vi "Add Elements to MeasLink UI.vi"(11 "error in (no error)":errorcluster) -> (15 "error out":errorcluster)   [LabVIEW 2021, in "Migrator.lvlib"]
uses:
  Migrator.lvlib
  Path Functions/Path Functions.lvlib
  Migrator Reusables/Migrator Reusables.lvlib
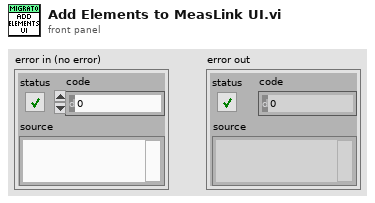
[diagram p1: front panel]
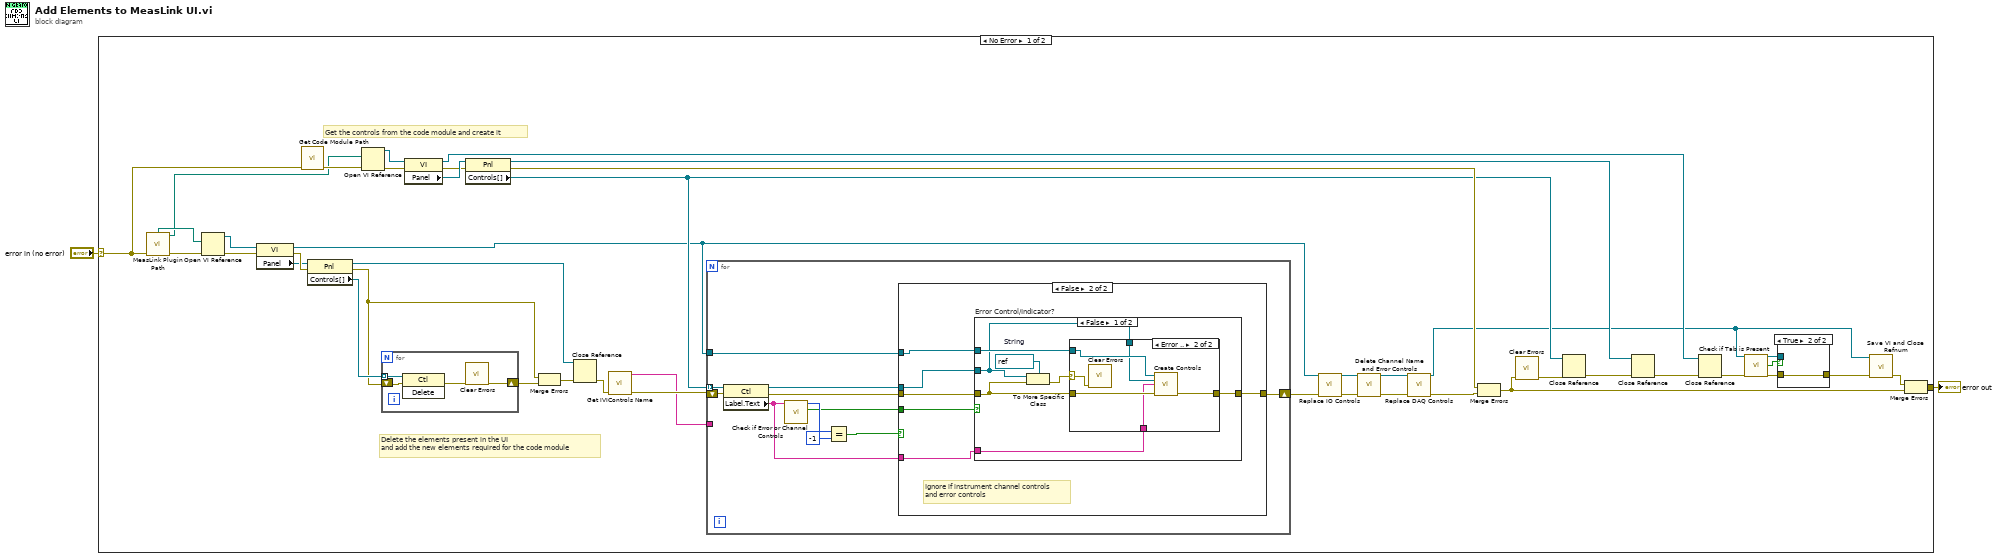
[diagram p0: block diagram]
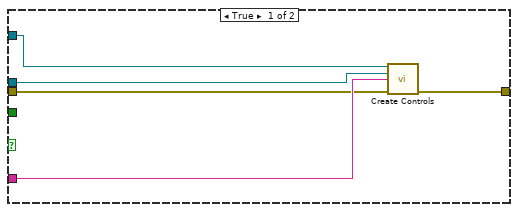
[diagram p2: hidden frame]
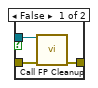
[diagram p5: hidden frame]
diagram:
  n1 = case shown="No Error" "error in (no error)" {
    selector: "error in (no error)" -> [w31 w92]
    tunnel: [w36 w92] -> w2
    frame No Error {
      # "Get the controls from the code module and create it"
      # "Delete the elements present in the UI\nand add the new elements required for the code module"
      n2 = call "MeasLink Plugin Path.vi"("error in (no error)"=w31) -> ("Measurement UI"=w33:path, "New Code Module"=w11:path, "error out"=w46:errorcluster)  [unwired: 2 in, 10 out]
      n3 = Open VI Reference(vi path=w33, error in (no error)=w46) -> (vi reference=w21:refnum<vi>, error out=w45:errorcluster)  [unwired: 4 in]
      n4 = property class="VI"(reference=w21, error in=w45) -> (reference out=w25:refnum<vi>, error out=w44:errorcluster, "Panel"=w27:refnum<vi>)
      n5 = call "Get Code Module Path.vi"("error in (no error)"=w31) -> ("error out"=w30:errorcluster)  [unwired: 13 in, 1 out]
      n6 = property class="Pnl"(reference=w27, error in=w44) -> (reference out=w26:refnum<vi>, error out=w12:errorcluster, "Controls[]"=w43:refnum<vi>[])
      n7 = Open VI Reference(vi path=w11, error in (no error)=w30) -> (vi reference=w18:refnum<vi>, error out=w38:errorcluster)  [unwired: 4 in]
      n8 = for {
        tunnel: w43 -> [w50] mode=indexing
        shift-right: [w47] -> w42
        shift-left: w12 -> [w49]
        n9 = invoke class="Ctl" method="Delete"(reference=w50, error in=w49) -> (error out=w48:errorcluster)  [unwired: 1 in, 2 out]
        n10 = call <vilib>:"Clear Errors.vi"("error in (no error)"=w48) -> ("error out"=w47:errorcluster)  [unwired: 5 in, 1 out]
      }
      n11 = property class="VI"(reference=w18, error in=w38) -> (reference out=w17:refnum<vi>, error out=w37:errorcluster, "Panel"=w39:refnum<vi>)
      n12 = property class="Pnl"(reference=w39, error in=w37) -> (reference out=w16:refnum<vi>, error out=w41:errorcluster, "Controls[]"=w40:refnum<vi>[])
      n13 = Merge Errors(w12, w42) -> (w13:errorcluster)
      n14 = Close Reference(reference=w26, error in (no error)=w13) -> (error out=w20:errorcluster)
      n15 = call "Get IVIControls Name.vi"("error in (no error)"=w20) -> ("Control Names Out"=w28:string[], "error out"=w29:errorcluster)  [unwired: 12 in, 1 out]
      n16 = for {
        tunnel: w25 -> [w61]
        tunnel: w40 -> [w59] mode=indexing
        shift-right: [w60] -> w24
        shift-left: w29 -> [w58]
        tunnel: w28 -> [_]
        n17 = property class="Ctl"(reference=w59, error in=w58) -> (reference out=w56:refnum<vi>, error out=w55:errorcluster, "Label.Text"=w57:string)
        n18 = call "Check if Error or Channel Controls.vi"("Label.Text"=w57) -> ("Error?"=w51:bool, "offset past match"=w54:i32)  [unwired: 9 in]
        n19 = Equal?(x=w54, y=-1) -> (x = y?=w52:bool)
        n20 = case shown="False" w52 {
          tunnel: w61 -> [w66 w69]
          tunnel: [w65 w67] -> w60
          tunnel: w56 -> [w63 w72]
          tunnel: w55 -> [w62 w71]
          tunnel: w57 -> [w64 w68]
          tunnel: w51 -> [_ w70]
          frame True {
            n21 = call "Create Controls.vi"("VI in"=w66, "Ctl Refnum"=w63, "Control Label"=w64, "error in (no error)"=w62) -> ("error out"=w65:errorcluster)  [unwired: 11 in]
          }
          frame False {
            # "Ignore if instrument channel controls\nand error controls"
            n22 = case "Error Control/Indicator?" shown="False" w70 {
              tunnel: w72 -> [w75 _]
              tunnel: w71 -> [w78 w87]
              tunnel: w69 -> [w76 _]
              tunnel: w68 -> [w74 _]
              tunnel: [w73 w87] -> w67
              frame False {
                w79 = refnum<vi> refnum  # String
                n23 = To More Specific Class(target class=w79, reference=w75, error in=w78) -> (error out=w77:errorcluster)  [unwired: 1 out]
                n24 = case shown="Error .." w77 {
                  selector: w77 -> [_ w81]
                  tunnel: w78 -> [w80 w86]
                  tunnel: w76 -> [_ w85]
                  tunnel: w75 -> [_ w84]
                  tunnel: w74 -> [_ w83]
                  tunnel: [w80 w82] -> w73
                  frame No Error {
                  }
                  frame Error {
                    n25 = call <vilib>:"Clear Errors.vi"("error in (no error)"=w81) -> ()  [unwired: 5 in, 2 out]
                    n26 = call "Create Controls.vi"("VI in"=w85, "Ctl Refnum"=w84, "Control Label"=w83, "error in (no error)"=w86) -> ("error out"=w82:errorcluster)  [unwired: 11 in]
                  }
                }
              }
              frame True {
              }
            }
          }
        }
      }
      n27 = call "Replace IO Controls.vi"("VI in"=w25, "error in (no error)"=w24) -> ("VI out"=w23:refnum<vi>, "error out"=w22:errorcluster)  [unwired: 12 in]
      n28 = call "Delete Channel Name and Error Controls.vi"("VI in"=w23, "error in (no error)"=w22) -> ("VI out"=w6:refnum<vi>, "error out"=w3:errorcluster)  [unwired: 12 in]
      n29 = call "Replace DAQ Controls.vi"("VI in"=w6, "error in (no error)"=w3) -> ("VI out"=w5:refnum<vi>, "error out"=w4:errorcluster)  [unwired: 12 in]
      n30 = Merge Errors(w41, w4) -> (w35:errorcluster)
      n31 = call <vilib>:"Clear Errors.vi"("error in (no error)"=w35) -> ("error out"=w34:errorcluster)  [unwired: 5 in, 1 out]
      n32 = Close Reference(reference=w40, error in (no error)=w34) -> (error out=w14:errorcluster)
      n33 = Close Reference(reference=w16, error in (no error)=w14) -> (error out=w15:errorcluster)
      n34 = Close Reference(reference=w17, error in (no error)=w15) -> (error out=w9:errorcluster)
      n35 = call "Check if Tab is Present.vi"("VI in"=w5, "error in (no error)"=w9) -> ("VI out"=w10:refnum<vi>, "Tab present?"=w7:bool, "error out"=w8:errorcluster)  [unwired: 11 in]
      n36 = case shown="True" w7 {
        tunnel: [w90 w91] -> w19
        tunnel: w10 -> [w89 _]
        tunnel: w8 -> [w88 w91]
        frame False {
          n37 = call "Call FP Cleanup.vi"("VI"=w89, "error in (no error)"=w88) -> ("error out"=w90:errorcluster)  [unwired: 13 in]
        }
        frame True {
        }
      }
      n38 = call "Save VI and Close Refnum.vi"("VI Refnum"=w5, "error in"=w19) -> ("error out"=w32:errorcluster)  [unwired: 13 in]
      n39 = Merge Errors(w32, w35) -> (w36:errorcluster)
    }
    frame Error {
    }
  }
  "error out" <- w2
